vi "Get Library Name.vi"(11 "error in (no error)":errorcluster) -> (4 "VI Path":path, 6 "Lib Name":string, 8 "VI Name":string, 15 "error out":errorcluster)   [LabVIEW 2021, in "G Plug-in Migrator.lvlib"]
uses:
  G Plug-in Migrator.lvlib
  Path Functions/Path Functions.lvlib
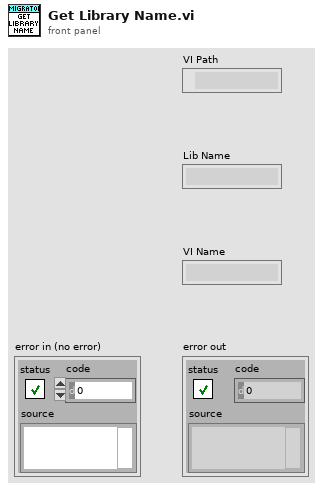
[diagram p1: front panel]
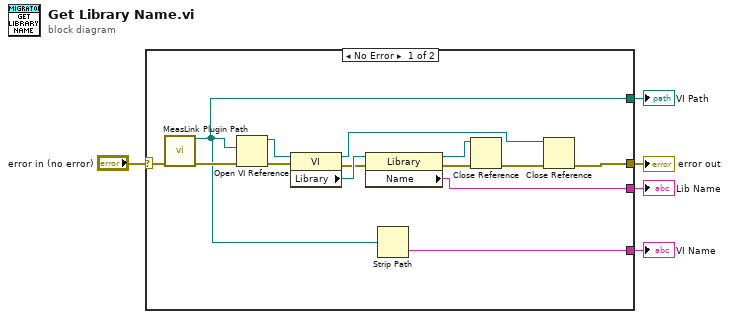
[diagram p0: block diagram]
diagram:
  n1 = case shown="No Error" "error in (no error)" {
    selector: "error in (no error)" -> [w19 w20]
    tunnel: [w8 w20] -> w5
    tunnel: [w9 _] -> w3
    tunnel: [w7 _] -> w2
    tunnel: [w6 _] -> w1
    frame No Error {
      n2 = call "MeasLink Plugin Path.vi"("error in (no error)"=w19) -> ("New Code Module"=w6:path, "error out"=w18:errorcluster)  [unwired: 2 in, 11 out]
      n3 = Open VI Reference(vi path=w6, error in (no error)=w18) -> (vi reference=w17:refnum<vi>, error out=w16:errorcluster)  [unwired: 4 in]
      n4 = property class="VI"(reference=w17, error in=w16) -> (reference out=w11:refnum<vi>, error out=w14:errorcluster, "Library"=w15:refnum<vi>)
      n5 = property class="Library"(reference=w15, error in=w14) -> (reference out=w12:refnum<vi>, error out=w13:errorcluster, "Name"=w9:string)
      n6 = Strip Path(path=w6) -> (name=w7:string)  [unwired: 1 out]
      n7 = Close Reference(reference=w12, error in (no error)=w13) -> (error out=w10:errorcluster)
      n8 = Close Reference(reference=w11, error in (no error)=w10) -> (error out=w8:errorcluster)
    }
    frame Error {
    }
  }
  "error out" <- w5
  "Lib Name" <- w3
  "VI Name" <- w2
  "VI Path" <- w1
